vi "test bool change.vi"() -> ()   [LabVIEW 2019]
uses:
  TypeDef/bool_data.ctl
  TypeDef/bool_setting.ctl
panel:
  out "delta iter 2":i32
  out "delta t ms 2":u32
  out "delta t ms":u32
  out "delta iter":i32
  out "Array in":bool[](array[boolean])
  out "Array out":bool[](array[boolean])
  in  "bool_setting":T1
  in  "bool_data_init":T2
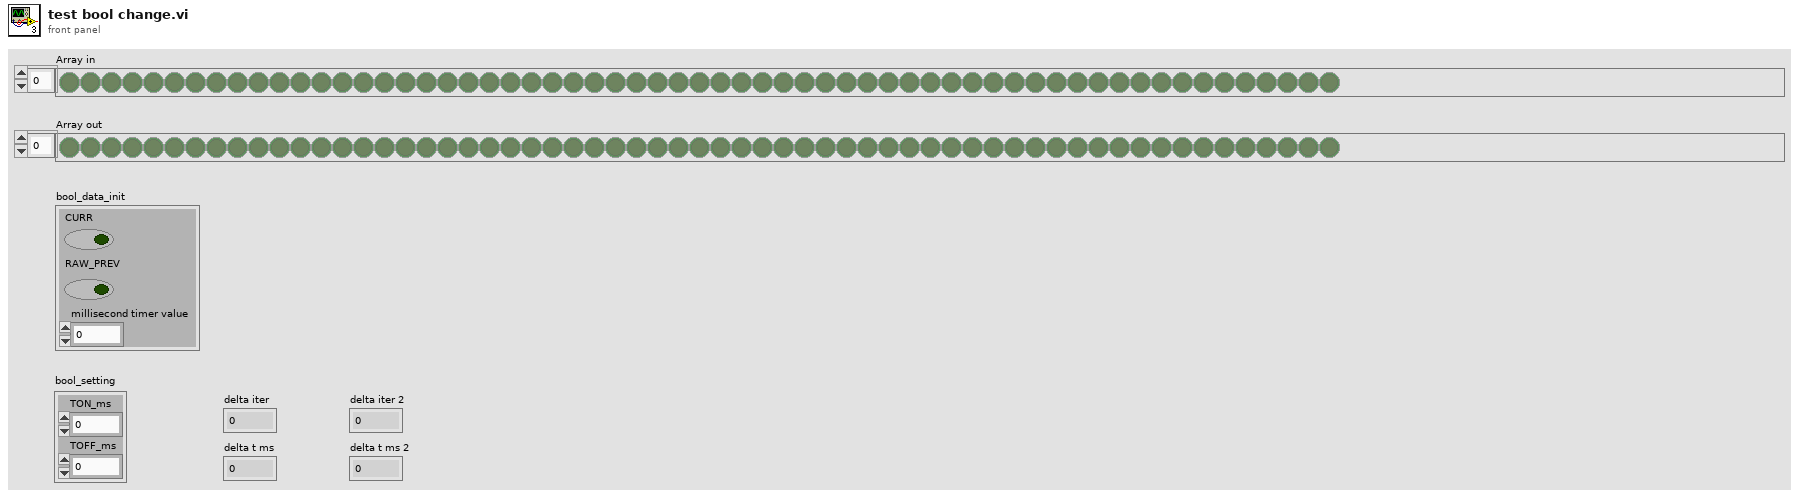
[diagram p1: front panel]
types:
  T1 = typedef "bool_setting.ctl" = cluster{"TON_ms":u32, "TOFF_ms":u32}
  T2 = typedef "bool_data.ctl" = cluster{"CURR":bool, "RAW_PREV":bool, "millisecond timer value":u32}
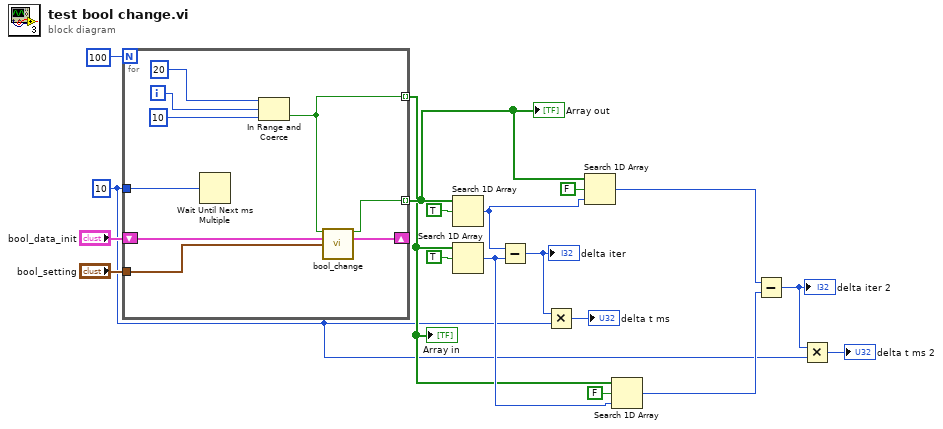
[diagram p0: block diagram]
diagram:
  w1 = u32 10 ("millisecond multiple")
  n1 = for {
    N: 100 -> [_]
    shift-right: [w27] -> _
    shift-left: "bool_data_init" -> [w26]
    tunnel: "bool_setting" -> [w25]
    tunnel: [w24] -> w11 mode=indexing
    tunnel: [w20] -> w6 mode=indexing
    tunnel: w1 -> [w23]
    i -> [w21]
    n2 = Wait Until Next ms Multiple(millisecond multiple=w23) -> ()  [unwired: 1 out]
    n3 = In Range and Coerce(upper limit=20, x=w21, lower limit=10 ("y")) -> (In Range?=w20:bool)  [unwired: 1 out]
    n4 = call "bool_change.vi"("RAW"=w20, "bool_data_in"=w26, "bool_setting"=w25) -> ("CURR"=w24:bool, "bool_data_out"=w27:T2)  [unwired: 11 in]
  }
  "Array out" <- w11
  "Array in" <- w6
  n5 = Search 1D Array(1D array=w11, element=TRUE) -> (index of element=w10:i32)  [unwired: 1 in]
  n6 = Search 1D Array(1D array=w6, element=TRUE) -> (index of element=w7:i32)  [unwired: 1 in]
  n7 = Subtract(x=w10, y=w7) -> (x-y=w13:i32)
  "delta iter" <- w13
  n8 = Multiply(x=w13, y=w1) -> (x*y=→"delta t ms":u32)
  n9 = Search 1D Array(1D array=w11, element=FALSE, start index (0)=w10) -> (index of element=w3:i32)
  n10 = Search 1D Array(1D array=w6, element=FALSE, start index (0)=w7) -> (index of element=w2:i32)
  n11 = Subtract(x=w3, y=w2) -> (x-y=w4:i32)
  "delta iter 2" <- w4
  n12 = Multiply(x=w4, y=w1) -> (x*y=→"delta t ms 2":u32)
